vi "RS_RF_query_LAN.vi"(1 "Parameter":T1(ring), 2 "IP address":string="0:19") -> (0 "value":dbl format="%#_24g")   [LabVIEW 2013]
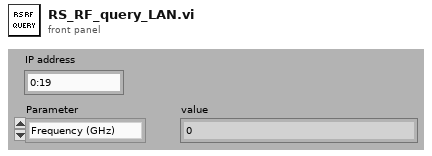
[diagram p1: front panel]
types:
  T1 = enum16{"Frequency (GHz)", "Power (dBm)", "Pulse period (us)", "Pulse width (us)", "Pulse delay (us)", "Pulse modulation?", "Output on?", "Pulse source", "Pulse mode", "Trigger mode", "Ex trigger input slope", "External impedance"}
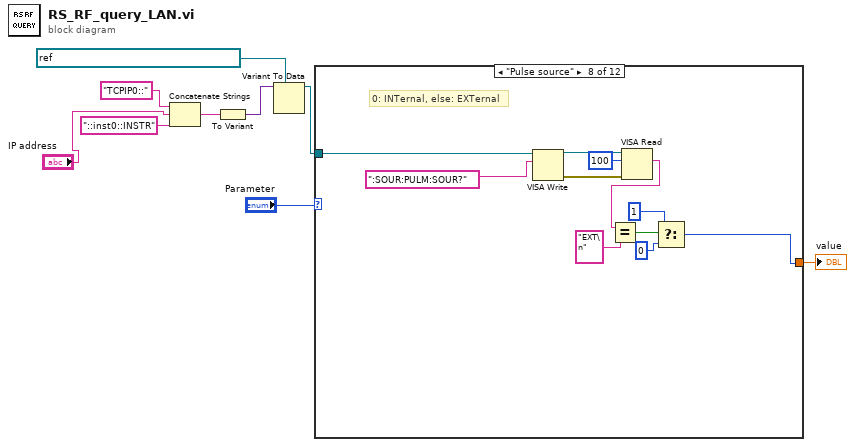
[diagram p0: block diagram]
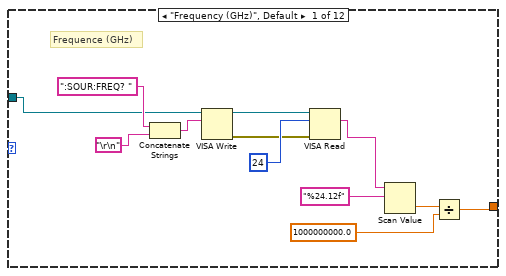
[diagram p2: hidden frame]
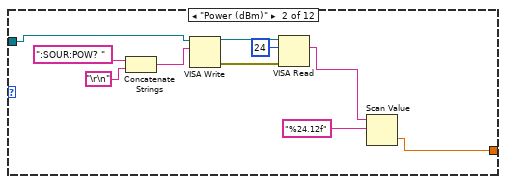
[diagram p3: hidden frame]
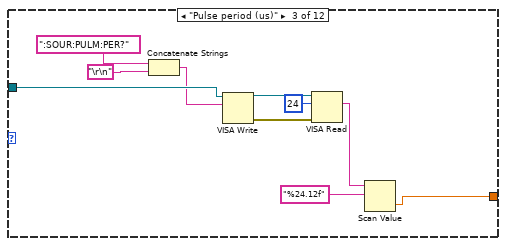
[diagram p4: hidden frame]
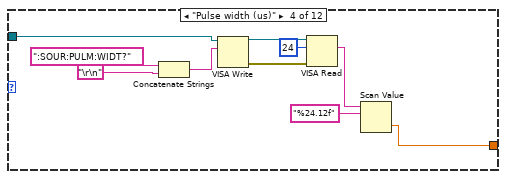
[diagram p5: hidden frame]
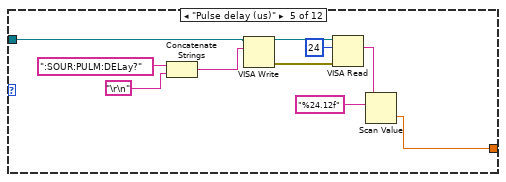
[diagram p6: hidden frame]
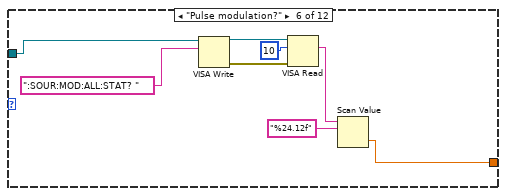
[diagram p7: hidden frame]
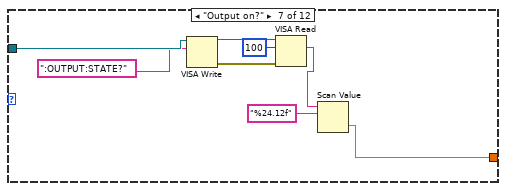
[diagram p8: hidden frame]
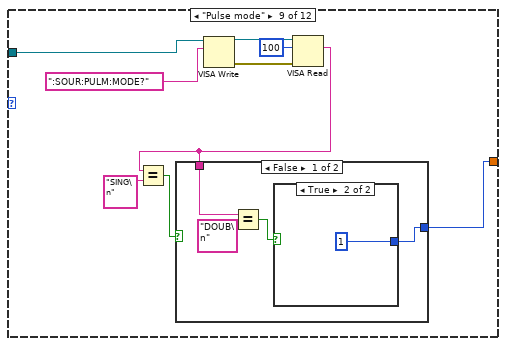
[diagram p9: hidden frame]
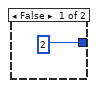
[diagram p10: hidden frame]
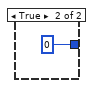
[diagram p11: hidden frame]
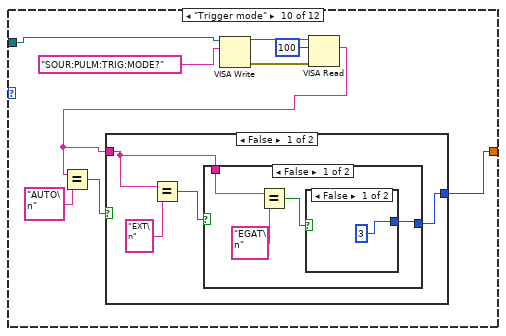
[diagram p12: hidden frame]
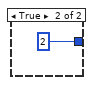
[diagram p13: hidden frame]
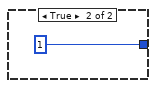
[diagram p14: hidden frame]
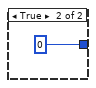
[diagram p15: hidden frame]
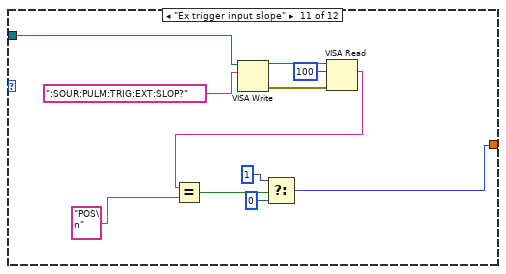
[diagram p16: hidden frame]
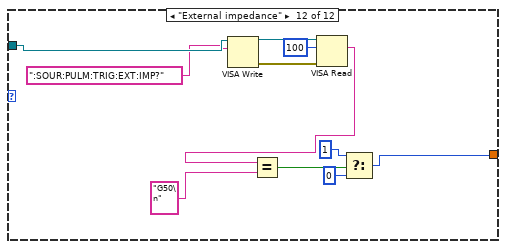
[diagram p17: hidden frame]
diagram:
  n1 = Concatenate Strings("TCPIP0::" ("string"), "IP address", "::inst0::INSTR" ("string")) -> (w7:string)
  n2 = To Variant(anything=w7) -> (Variant=w4:variant)
  n3 = Variant To Data(type=refnum<visa-resource-name> "visa://192.168.137.11/RIO0::INSTR" ("VISA resource name"), Variant=w4) -> (data=w1:refnum<visa-resource-name>)  [unwired: 1 in, 1 out]
  n4 = case shown="\"Pulse source\"" "Parameter" {
    tunnel: w1 -> [w14 w24 w34 w44 w54 w64 w72 w81 w91 w107 w128 w139]
    tunnel: [w16 w28 w38 w48 w58 w68 w76 w85 w95 w111 w132 w143] -> w8
    frame "Frequency (GHz)", Default {
      # "Frequence (GHz)"
      n5 = Concatenate Strings(":SOUR:FREQ? " ("string"), "\r\n") -> (w19:string)
      n6 = VISA Write(VISA resource name=w14, write buffer=w19) -> (VISA resource name out=w10:refnum<visa-resource-name>, error out=w11:errorcluster)  [unwired: 1 in, 1 out]
      n7 = VISA Read(VISA resource name=w10, byte count=24, error in (no error)=w11) -> (read buffer=w12:string)  [unwired: 3 out]
      n8 = Scan Value(string=w12, format string="%24.12f") -> (value=w17:dbl)  [unwired: 1 in, 1 out]
      n9 = Divide(x=w17, y=1000000000.0) -> (x/y=w16:dbl)
    }
    frame "Power (dBm)" {
      n10 = Concatenate Strings(":SOUR:POW? " ("string"), "\r\n") -> (w23:string)
      n11 = VISA Write(VISA resource name=w24, write buffer=w23) -> (VISA resource name out=w25:refnum<visa-resource-name>, error out=w26:errorcluster)  [unwired: 1 in, 1 out]
      n12 = VISA Read(VISA resource name=w25, byte count=u32 24, error in (no error)=w26) -> (read buffer=w22:string)  [unwired: 3 out]
      n13 = Scan Value(string=w22, format string="%24.12f") -> (value=w28:dbl)  [unwired: 1 in, 1 out]
    }
    frame "Pulse period (us)" {
      n14 = Concatenate Strings(":SOUR:PULM:PER?" ("string"), "\r\n") -> (w33:string)
      n15 = VISA Write(VISA resource name=w34, write buffer=w33) -> (VISA resource name out=w35:refnum<visa-resource-name>, error out=w36:errorcluster)  [unwired: 1 in, 1 out]
      n16 = VISA Read(VISA resource name=w35, byte count=u32 24, error in (no error)=w36) -> (read buffer=w32:string)  [unwired: 3 out]
      n17 = Scan Value(string=w32, format string="%24.12f") -> (value=w38:dbl)  [unwired: 1 in, 1 out]
    }
    frame "Pulse width (us)" {
      n18 = Concatenate Strings(":SOUR:PULM:WIDT?" ("string"), "\r\n") -> (w43:string)
      n19 = VISA Write(VISA resource name=w44, write buffer=w43) -> (VISA resource name out=w45:refnum<visa-resource-name>, error out=w46:errorcluster)  [unwired: 1 in, 1 out]
      n20 = VISA Read(VISA resource name=w45, byte count=u32 24, error in (no error)=w46) -> (read buffer=w42:string)  [unwired: 3 out]
      n21 = Scan Value(string=w42, format string="%24.12f") -> (value=w48:dbl)  [unwired: 1 in, 1 out]
    }
    frame "Pulse delay (us)" {
      n22 = Concatenate Strings(":SOUR:PULM:DELay?" ("string"), "\r\n") -> (w53:string)
      n23 = VISA Write(VISA resource name=w54, write buffer=w53) -> (VISA resource name out=w55:refnum<visa-resource-name>, error out=w56:errorcluster)  [unwired: 1 in, 1 out]
      n24 = VISA Read(VISA resource name=w55, byte count=u32 24, error in (no error)=w56) -> (read buffer=w52:string)  [unwired: 3 out]
      n25 = Scan Value(string=w52, format string="%24.12f") -> (value=w58:dbl)  [unwired: 1 in, 1 out]
    }
    frame "Pulse modulation?" {
      n26 = VISA Write(VISA resource name=w64, write buffer=":SOUR:MOD:ALL:STAT? " ("string")) -> (VISA resource name out=w65:refnum<visa-resource-name>, error out=w66:errorcluster)  [unwired: 1 in, 1 out]
      n27 = VISA Read(VISA resource name=w65, byte count=u32 10, error in (no error)=w66) -> (read buffer=w62:string)  [unwired: 3 out]
      n28 = Scan Value(string=w62, format string="%24.12f") -> (value=w68:dbl)  [unwired: 1 in, 1 out]
    }
    frame "Output on?" {
      n29 = VISA Write(VISA resource name=w72, write buffer=":OUTPUT:STATE?") -> (VISA resource name out=w73:refnum<visa-resource-name>, error out=w74:errorcluster)  [unwired: 1 in, 1 out]
      n30 = VISA Read(VISA resource name=w73, byte count=u32 100, error in (no error)=w74) -> (read buffer=w70:string)  [unwired: 3 out]
      n31 = Scan Value(string=w70, format string="%24.12f") -> (value=w76:dbl)  [unwired: 1 in, 1 out]
    }
    frame "Pulse source" {
      # "0: INTernal, else: EXTernal"
      n32 = VISA Write(VISA resource name=w81, write buffer=":SOUR:PULM:SOUR?") -> (VISA resource name out=w82:refnum<visa-resource-name>, error out=w83:errorcluster)  [unwired: 1 in, 1 out]
      n33 = VISA Read(VISA resource name=w82, byte count=u32 100, error in (no error)=w83) -> (read buffer=w79:string)  [unwired: 3 out]
      n34 = Equal?(x=w79, y="EXT\n") -> (x = y?=w88:bool)
      n35 = Select(t=1, s=w88, f=0) -> (s? t:f=w85:i32)
    }
    frame "Pulse mode" {
      n36 = VISA Write(VISA resource name=w91, write buffer=":SOUR:PULM:MODE?") -> (VISA resource name out=w92:refnum<visa-resource-name>, error out=w93:errorcluster)  [unwired: 1 in, 1 out]
      n37 = VISA Read(VISA resource name=w92, byte count=u32 100, error in (no error)=w93) -> (read buffer=w89:string)  [unwired: 3 out]
      n38 = Equal?(x=w89, y="SING\n") -> (x = y?=w96:bool)
      n39 = case shown="False" w96 {
        tunnel: [w98 0] -> w95
        tunnel: w89 -> [w100 _]
        frame False {
          n40 = Equal?(x=w100, y="DOUB\n") -> (x = y?=w99:bool)
          n41 = case shown="True" w99 {
            tunnel: [2 1] -> w98
            frame False {
            }
            frame True {
            }
          }
        }
        frame True {
        }
      }
    }
    frame "Trigger mode" {
      n42 = VISA Write(VISA resource name=w107, write buffer="SOUR:PULM:TRIG:MODE?") -> (VISA resource name out=w108:refnum<visa-resource-name>, error out=w109:errorcluster)  [unwired: 1 in, 1 out]
      n43 = VISA Read(VISA resource name=w108, byte count=u32 100, error in (no error)=w109) -> (read buffer=w105:string)  [unwired: 3 out]
      n44 = Equal?(x=w105, y="AUTO\n") -> (x = y?=w112:bool)
      n45 = case shown="False" w112 {
        tunnel: w105 -> [w114 _]
        tunnel: [w115 0] -> w111
        frame False {
          n46 = Equal?(x=w114, y="EXT\n") -> (x = y?=w116:bool)
          n47 = case shown="False" w116 {
            tunnel: [w118 1] -> w115
            tunnel: w114 -> [w120 _]
            frame False {
              n48 = Equal?(x=w120, y="EGAT\n") -> (x = y?=w119:bool)
              n49 = case shown="False" w119 {
                tunnel: [3 2] -> w118
                frame False {
                }
                frame True {
                }
              }
            }
            frame True {
            }
          }
        }
        frame True {
        }
      }
    }
    frame "Ex trigger input slope" {
      n50 = VISA Write(VISA resource name=w128, write buffer=":SOUR:PULM:TRIG:EXT:SLOP?") -> (VISA resource name out=w129:refnum<visa-resource-name>, error out=w130:errorcluster)  [unwired: 1 in, 1 out]
      n51 = VISA Read(VISA resource name=w129, byte count=u32 100, error in (no error)=w130) -> (read buffer=w126:string)  [unwired: 3 out]
      n52 = Equal?(x=w126, y="POS\n") -> (x = y?=w135:bool)
      n53 = Select(t=1, s=w135, f=0) -> (s? t:f=w132:i32)
    }
    frame "External impedance" {
      n54 = VISA Write(VISA resource name=w139, write buffer=":SOUR:PULM:TRIG:EXT:IMP?") -> (VISA resource name out=w140:refnum<visa-resource-name>, error out=w141:errorcluster)  [unwired: 1 in, 1 out]
      n55 = VISA Read(VISA resource name=w140, byte count=u32 100, error in (no error)=w141) -> (read buffer=w137:string)  [unwired: 3 out]
      n56 = Equal?(x=w137, y="G50\n") -> (x = y?=w146:bool)
      n57 = Select(t=1, s=w146, f=0) -> (s? t:f=w143:i32)
    }
  }
  "value" <- w8
